vi "Multimètre.vi"(2 "Commande":string, 3 "Ressource GPIB VISA":refnum<visa-resource-name>="GPIB0::2::INSTR") -> (0 "tension en chaine de caractères":string)   [LabVIEW 2024]
panel:
  out "Tension relevée":dbl(knob) scale=-9e-10..0.01
  in  "Waveform":enum16{"SIN", "SQU", "RAND"}(ring)
  out "Données brutes":string
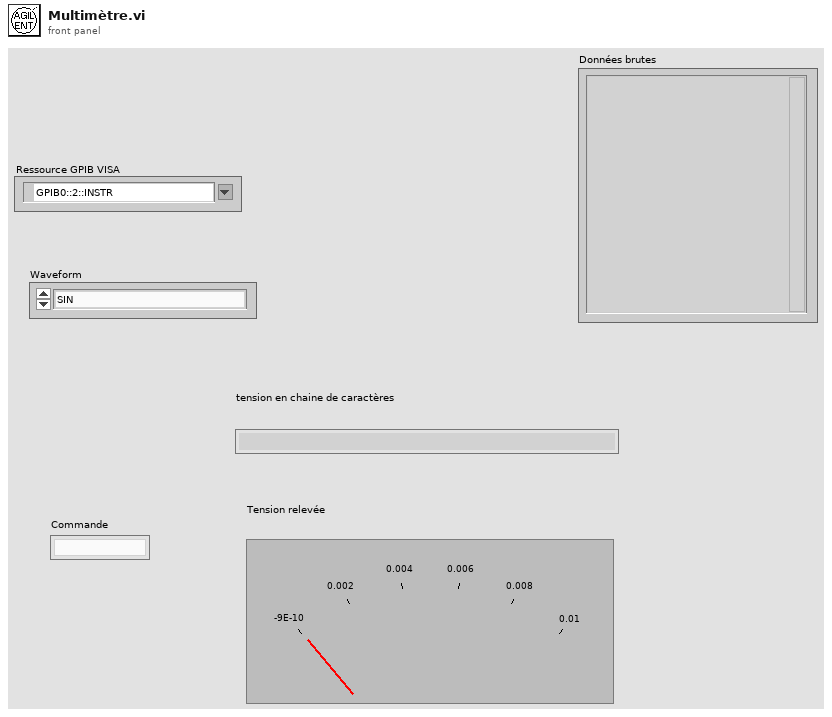
[diagram p1: front panel]
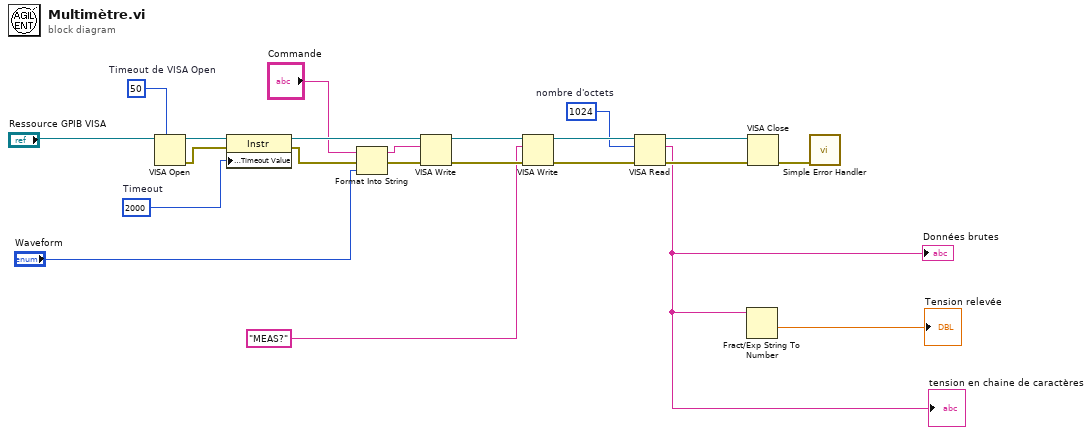
[diagram p0: block diagram]
diagram:
  w14 = u32 1024  # nombre d'octets
  w17 = u32 2000  # Timeout
  w18 = u32 50  # Timeout de VISA Open
  n1 = VISA Open(timeout (0)=w18, VISA resource name="Ressource GPIB VISA") -> (VISA resource name=w16:refnum<visa-resource-name>, error out=w15:errorcluster)  [unwired: 3 in]
  n2 = property class="Instr"(reference=w16, error in=w15, "General Settings:Timeout Value"=w17) -> (reference out=w12:refnum<visa-resource-name>, error out=w9:errorcluster)
  n3 = Format Into String(initial string="Commande", error in=w9, "Waveform") -> (resulting string=w7:string, error out=w8:errorcluster)  [unwired: 1 in]
  n4 = VISA Write(VISA resource name=w12, write buffer=w7, error in (no error)=w8) -> (VISA resource name out=w11:refnum<visa-resource-name>, error out=w10:errorcluster)  [unwired: 1 out]
  n5 = VISA Write(VISA resource name=w11, write buffer="MEAS?", error in (no error)=w10) -> (VISA resource name out=w22:refnum<visa-resource-name>, error out=w20:errorcluster)  [unwired: 1 out]
  n6 = VISA Read(VISA resource name=w22, byte count=w14, error in (no error)=w20) -> (VISA resource name out=w21:refnum<visa-resource-name>, read buffer=w2:string, error out=w19:errorcluster)  [unwired: 1 out]
  "Données brutes" <- w2
  "tension en chaine de caractères" <- w2
  n7 = Fract/Exp String To Number(string=w2) -> (number=→"Tension relevée":dbl)  [unwired: 3 in, 1 out]
  n8 = VISA Close(VISA resource name=w21, error in (no error)=w19) -> (error out=w13:errorcluster)
  n9 = call <vilib>:"Simple Error Handler.vi"("error in (no error)"=w13) -> ()  [unwired: 4 in, 5 out]
